vi "CheckForExit.vi"(8 "Name":string) -> (2 "Name out":string, 4 "exit":bool)   [LabVIEW 2014, in "SimpleMessaging.lvlib"]
uses:
  SimpleMessaging.lvlib
panel:
  in  "exit name ('exit')":string="exit"
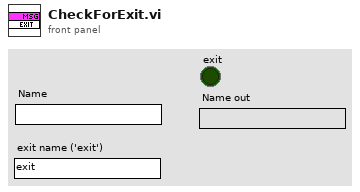
[diagram p1: front panel]
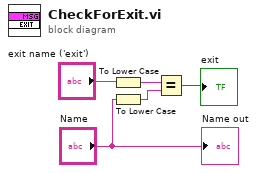
[diagram p0: block diagram]
diagram:
  n1 = To Lower Case(string="exit name ('exit')") -> (all lower case string=w3:string)
  n2 = To Lower Case(string="Name") -> (all lower case string=w2:string)
  n3 = Equal?(x=w3, y=w2) -> (x = y?=→"exit":bool)
  "Name out" <- "Name"
